vi "GOOP_VI_Item_OnCommand.vi"(10 "Command Tag":string, 11 "Object":u64) -> ()   [LabVIEW 2020]
uses:
  SubVIs/GOOP_ClassProviderClassType.ctl
  ClassProviders/Provider_BaseClassInterface/ClassWriter_class/ClassWriter.lvclass
  SubVIs/GOOP_UMLEditor_CallMainAction.ctl
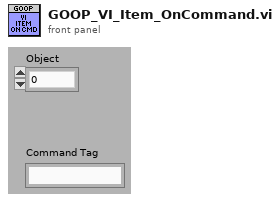
[diagram p1: front panel]
types:
  T1 = typedef "GOOP_ClassProviderClassType.ctl" = enum16{"ClassWriter", "ClassReader"}
  T2 = typedef "GOOP_UMLEditor_CallMainAction.ctl" = enum16{"OpenUmlEditor", "ReverseEngineering:WholeProject", "ReverseEngineering:OneClass", "ReverseEngineering:OneVI", "ShowInStateDiagram:OneVI", "OpenUMLFile"}
  T3 = typedef "ClassWriter.lvclass/RenameViOption.ctl" = cluster{"NewVIName":string, "VIs":path[], "IconOut":u8[][], "BgColor":u8}
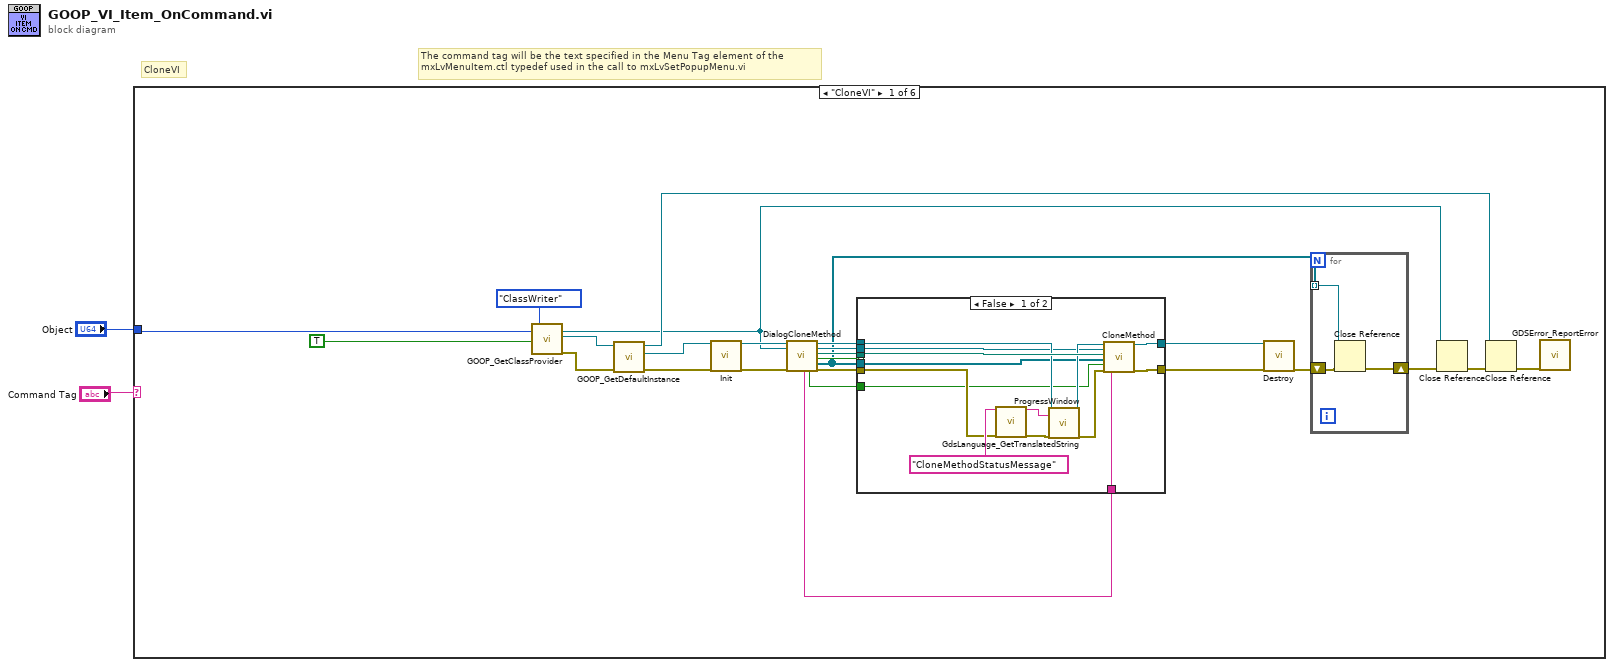
[diagram p0: block diagram]
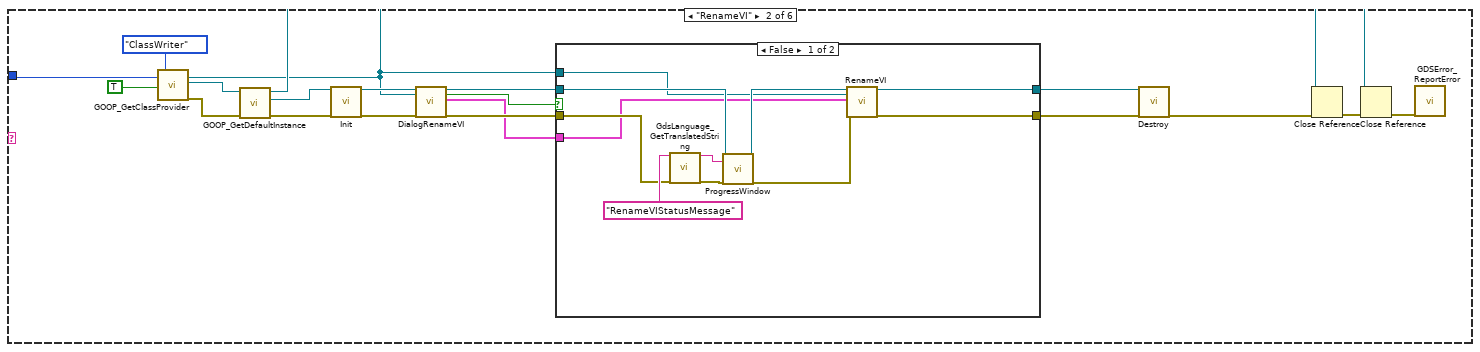
[diagram p3: hidden frame]
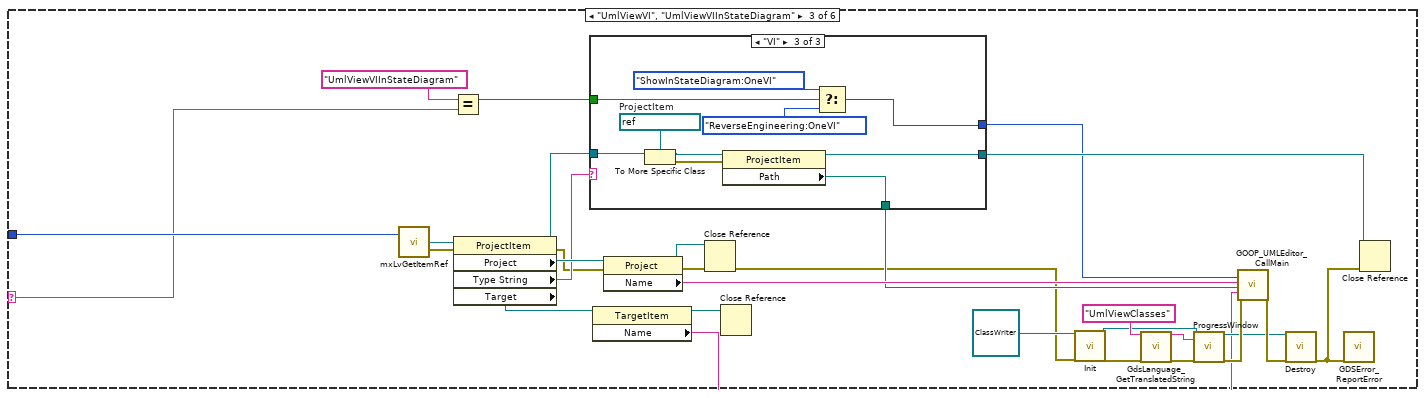
[diagram p5: hidden frame]
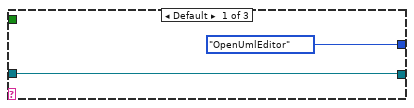
[diagram p6: hidden frame]
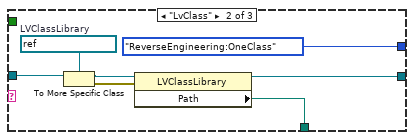
[diagram p7: hidden frame]
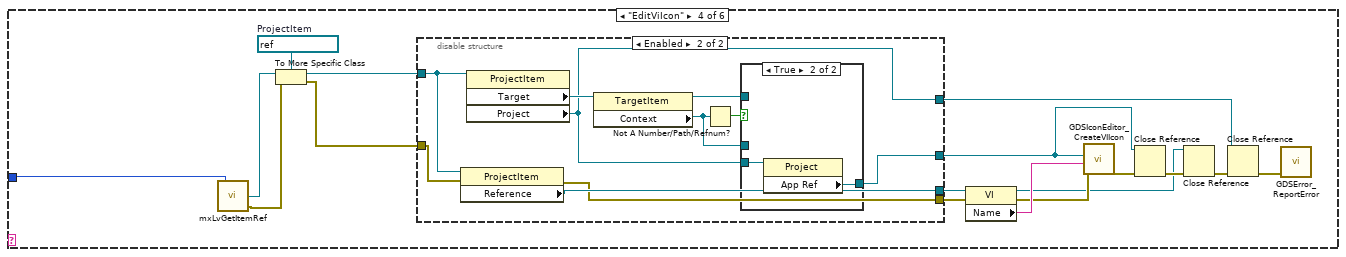
[diagram p8: hidden frame]
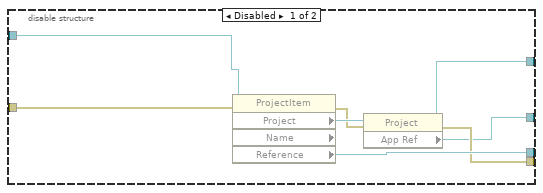
[diagram p9: hidden frame]
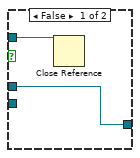
[diagram p10: hidden frame]
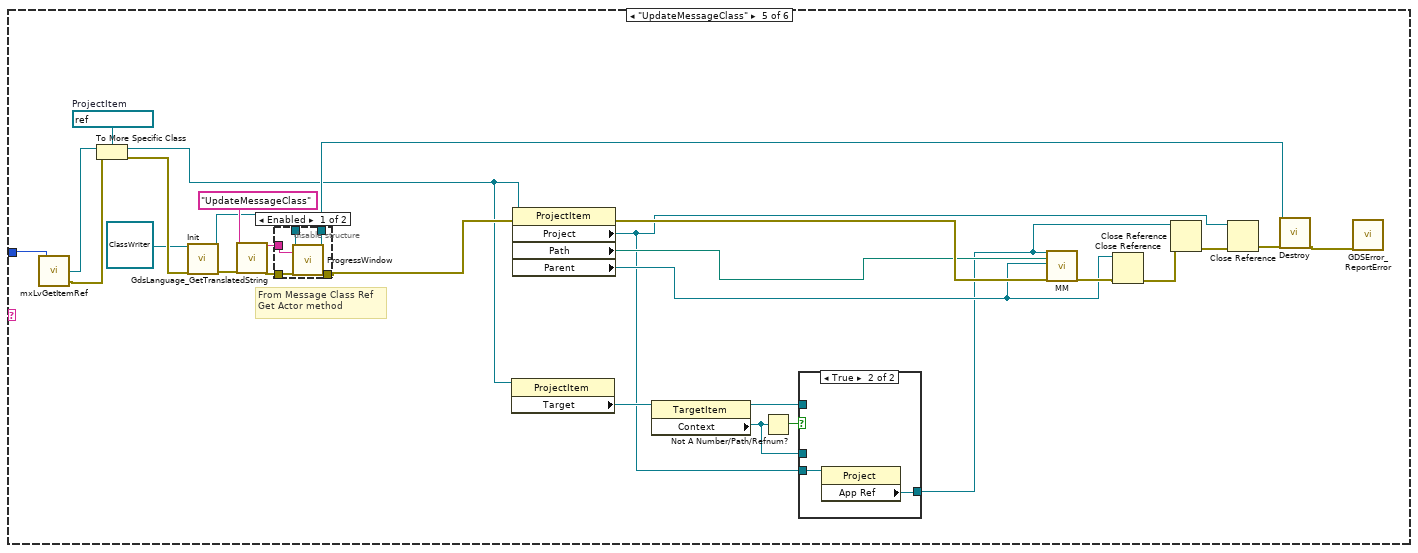
[diagram p11: hidden frame]
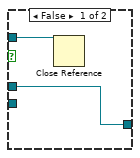
[diagram p12: hidden frame]
diagram:
  # "CloneVI"
  # "The command tag will be the text specified in the Menu Tag element of the \nmxLvMenuItem.ctl typedef used in the call to mxLvSetPopupMenu.vi"
  n1 = case shown="\"CloneVI\"" "Command Tag" {
    selector: "Command Tag" -> [_ _ w87 _ _ _]
    tunnel: "Object" -> [w24 w63 w89 w143 w193 _]
    frame "CloneVI" {
      n2 = call "GOOP_GetClassProvider.vi"("New Item Parent/Object"=w24, "CreateClass"=TRUE, "ProviderClassType"=GOOP_ClassProviderClassType."ClassWriter") -> ("ProjectItem"=w9:refnum<vi>, "LVClass.Open"=w22:refnum<vi>, "error out"=w23:errorcluster)  [unwired: 14 in]
      n3 = call "GOOP_GetDefaultInstance.vi"("error in"=w23, "LVClassIn"=w22) -> ("error out"=w20:errorcluster, "ClassWriter.lvclass"=w21:refnum<class "ClassWriter.lvclass">, "LVClassOut"=w19:refnum<vi>)  [unwired: 7 in]
      n4 = call-dynamic "Init.vi"("ClassWriter in"=w21, "error in (no error)"=w20) -> ("ClassWriter out"=w26:refnum<class "ClassWriter.lvclass">, "error out"=w25:errorcluster)  [unwired: 16 in]
      n5 = call-dynamic "DialogCloneMethod.vi"("ClassWriter.lvclass"=w26, "VIItemRefIn"=w9, "error in (no error)"=w25) -> ("NewVIDescriptionOut"=w3:string, "OpenAfter"=w4:bool, "ClassWriter.lvclassOut"=w17:refnum<class "ClassWriter.lvclass">, "VIItemRefOut"=w11:refnum<vi>, "NewVIPath"=w13:path, "Cancelled"=w14:bool, "LibraryOwners"=w6:refnum<vi>[], "error out"=w16:errorcluster)  [unwired: 9 in]
      n6 = case shown="False" w14 {
        tunnel: w17 -> [w37 w45]
        tunnel: w16 -> [w38 w46]
        tunnel: [w42 w46] -> w15
        tunnel: w13 -> [w44 _]
        tunnel: [w43 w45] -> w12
        tunnel: w6 -> [w34 _]
        tunnel: w11 -> [w33 _]
        tunnel: w4 -> [w32 _]
        tunnel: w3 -> [w31 _]
        frame False {
          n7 = call "GdsLanguage_GetTranslatedString.vi"("StringID(s)"="CloneMethodStatusMessage" ("Message(Exit)"), "error in (no error)"=w38) -> ("FirstStringOut"=w39:string, "error out"=w40:errorcluster)  [unwired: 14 in, 2 out]
          n8 = call-dynamic "ProgressWindow.vi"("ClassWriter in"=w37, "Message(Exit)"=w39, "error in (no error)"=w40) -> ("ClassWriter out"=w36:refnum<class "ClassWriter.lvclass">, "error out"=w35:errorcluster)  [unwired: 15 in]
          n9 = call-dynamic "CloneMethod.vi"("ClassWriter.lvclass"=w36, "VIItemRefIn"=w33, "NewVIPath"=w44, "LibraryOwners"=w34, "OpenVIWhenDone"=w32, "error in (no error)"=w35, "ViDescription"=w31) -> ("ClassWriter.lvclass"=w43:refnum<class "ClassWriter.lvclass">, "error out"=w42:errorcluster)  [unwired: 11 in]
        }
        frame True {
        }
      }
      n10 = call-dynamic "Destroy.vi"("ClassWriter.lvclass"=w12, "error in (no error)"=w15) -> ("error out"=w8:errorcluster)  [unwired: 17 in]
      n11 = for {
        shift-right: [w29] -> w7
        shift-left: w8 -> [w30]
        tunnel: w6 -> [w28] mode=indexing
        n12 = Close Reference(reference=w28, error in (no error)=w30) -> (error out=w29:errorcluster)
      }
      n13 = Close Reference(reference=w9, error in (no error)=w7) -> (error out=w10:errorcluster)
      n14 = Close Reference(reference=w19, error in (no error)=w10) -> (error out=w5:errorcluster)
      n15 = call "GDSError_ReportError.vi"("error in (no error)"=w5) -> ()  [unwired: 18 in, 1 out]
    }
    frame "RenameVI" {
      n16 = call "GOOP_GetClassProvider.vi"("New Item Parent/Object"=w63, "CreateClass"=TRUE, "ProviderClassType"=GOOP_ClassProviderClassType."ClassWriter") -> ("ProjectItem"=w47:refnum<vi>, "LVClass.Open"=w61:refnum<vi>, "error out"=w62:errorcluster)  [unwired: 14 in]
      n17 = call "GOOP_GetDefaultInstance.vi"("error in"=w62, "LVClassIn"=w61) -> ("error out"=w59:errorcluster, "ClassWriter.lvclass"=w60:refnum<class "ClassWriter.lvclass">, "LVClassOut"=w58:refnum<vi>)  [unwired: 7 in]
      n18 = call-dynamic "Init.vi"("ClassWriter in"=w60, "error in (no error)"=w59) -> ("ClassWriter out"=w65:refnum<class "ClassWriter.lvclass">, "error out"=w64:errorcluster)  [unwired: 16 in]
      n19 = call-dynamic "DialogRenameVI.vi"("ClassWriter.lvclass"=w65, "VIItemRefIn"=w47, "error in (no error)"=w64) -> ("ClassWriter.lvclassOut"=w56:refnum<class "ClassWriter.lvclass">, "Cancelled"=w49:bool, "RenameOption"=w48:T3, "error out"=w55:errorcluster)  [unwired: 13 in]
      n20 = case shown="False" w49 {
        tunnel: w56 -> [w71 w78]
        tunnel: w55 -> [w72 w79]
        tunnel: [w76 w79] -> w54
        tunnel: [w77 w78] -> w53
        tunnel: w48 -> [w67 _]
        tunnel: w47 -> [w68 _]
        frame False {
          n21 = call "GdsLanguage_GetTranslatedString.vi"("StringID(s)"="RenameVIStatusMessage" ("Message(Exit)"), "error in (no error)"=w72) -> ("FirstStringOut"=w73:string, "error out"=w74:errorcluster)  [unwired: 14 in, 2 out]
          n22 = call-dynamic "ProgressWindow.vi"("ClassWriter in"=w71, "Message(Exit)"=w73, "error in (no error)"=w74) -> ("ClassWriter out"=w70:refnum<class "ClassWriter.lvclass">, "error out"=w69:errorcluster)  [unwired: 15 in]
          n23 = call-dynamic "RenameVI.vi"("ObjectIn"=w70, "VIItemRefIn"=w68, "RenameOption"=w67, "error in (no error)"=w69) -> ("ObjectOut"=w77:refnum<class "ClassWriter.lvclass">, "error out"=w76:errorcluster)  [unwired: 14 in]
        }
        frame True {
        }
      }
      n24 = call-dynamic "Destroy.vi"("ClassWriter.lvclass"=w53, "error in (no error)"=w54) -> ("error out"=w51:errorcluster)  [unwired: 17 in]
      n25 = Close Reference(reference=w47, error in (no error)=w51) -> (error out=w52:errorcluster)
      n26 = Close Reference(reference=w58, error in (no error)=w52) -> (error out=w50:errorcluster)
      n27 = call "GDSError_ReportError.vi"("error in (no error)"=w50) -> ()  [unwired: 18 in, 1 out]
    }
    frame "UmlViewVI", "UmlViewVIInStateDiagram" {
      n28 = call <resource>:"mxLvGetItemRef.vi"("Item"=w89) -> ("Item Refnum"=w109:refnum<vi>, "error out"=w99:errorcluster)  [unwired: 1 in, 1 out]
      n29 = Equal?(x="UmlViewVIInStateDiagram", y=w87) -> (x = y?=w85:bool)
      n30 = property class="ProjectItem"(reference=w109, error in=w99) -> (reference out=w104:refnum<vi>, error out=w100:errorcluster, "Project"=w108:refnum<vi>, "Type String"=w102:string, "Target"=w81:refnum<vi>)
      n31 = case shown="\"VI\"" w102 {
        tunnel: w104 -> [w111 w118 w128]
        tunnel: [w111 w114 w124] -> w103
        tunnel: [_ w113 w123] -> w101
        tunnel: [GOOP_UMLEditor_CallMainAction."OpenUmlEditor" ("Enum") GOOP_UMLEditor_CallMainAction."ReverseEngineering:OneClass" ("Enum") w119] -> w88
        tunnel: w85 -> [_ _ w122]
        frame Default {
        }
        frame "LvClass" {
          w117 = refnum<vi> refnum  # LVClassLibrary
          n32 = To More Specific Class(target class=w117, reference=w118) -> (specific class reference=w116:refnum<vi>, error out=w115:errorcluster)  [unwired: 1 in]
          n33 = property class="LVClassLibrary"(reference=w116, error in=w115) -> (reference out=w114:refnum<vi>, "Path"=w113:path)  [unwired: 1 out]
        }
        frame "VI" {
          w127 = refnum<vi> refnum  # ProjectItem
          n34 = To More Specific Class(target class=w127, reference=w128) -> (specific class reference=w126:refnum<vi>, error out=w125:errorcluster)  [unwired: 1 in]
          n35 = property class="ProjectItem"(reference=w126, error in=w125) -> (reference out=w124:refnum<vi>, "Path"=w123:path)  [unwired: 1 out]
          n36 = Select(t=GOOP_UMLEditor_CallMainAction."ShowInStateDiagram:OneVI" ("Enum"), s=w122, f=GOOP_UMLEditor_CallMainAction."ReverseEngineering:OneVI" ("Enum")) -> (s? t:f=w119:T2)
        }
      }
      n37 = property class="TargetItem"(reference=w81) -> (reference out=w82:refnum<vi>, "Name"=w80:string)  [unwired: 1 in, 1 out]
      n38 = property class="Project"(reference=w108, error in=w100) -> (reference out=w105:refnum<vi>, error out=w106:errorcluster, "Name"=w107:string)
      n39 = Close Reference(reference=w105, error in (no error)=w106) -> (error out=w83:errorcluster)
      n40 = Close Reference(reference=w82) -> ()  [unwired: 1 in, 1 out]
      n41 = call-dynamic "Init.vi"("ClassWriter in"=refnum<class "ClassWriter.lvclass"> refnum, "error in (no error)"=w83) -> ("ClassWriter out"=w91:refnum<class "ClassWriter.lvclass">, "error out"=w95:errorcluster)  [unwired: 16 in]
      n42 = call "GdsLanguage_GetTranslatedString.vi"("StringID(s)"="UmlViewClasses" ("Message(Exit)"), "error in (no error)"=w95) -> ("FirstStringOut"=w98:string, "error out"=w97:errorcluster)  [unwired: 14 in, 2 out]
      n43 = call-dynamic "ProgressWindow.vi"("ClassWriter in"=w91, "Message(Exit)"=w98, "error in (no error)"=w97) -> ("ClassWriter out"=w92:refnum<class "ClassWriter.lvclass">, "error out"=w94:errorcluster)  [unwired: 15 in]
      n44 = call "GOOP_UMLEditor_CallMain.vi"("Enum"=w88, "Project"=w107, "Class/VI-Path"=w101, "Target"=w80, "error in (no error)"=w94) -> ("error out"=w93:errorcluster)  [unwired: 14 in]
      n45 = call-dynamic "Destroy.vi"("ClassWriter.lvclass"=w92, "error in (no error)"=w93) -> ("error out"=w84:errorcluster)  [unwired: 17 in]
      n46 = call "GDSError_ReportError.vi"("error in (no error)"=w84) -> ()  [unwired: 18 in, 1 out]
      n47 = Close Reference(reference=w103, error in (no error)=w84) -> ()  [unwired: 1 out]
    }
    frame "EditViIcon" {
      w145 = refnum<vi> refnum  # ProjectItem
      n48 = call <resource>:"mxLvGetItemRef.vi"("Item"=w143) -> ("Item Refnum"=w144:refnum<vi>, "error out"=w139:errorcluster)  [unwired: 1 in, 1 out]
      n49 = To More Specific Class(target class=w145, reference=w144, error in=w139) -> (specific class reference=w130:refnum<vi>, error out=w140:errorcluster)
      n50 = disable-structure shown="Enabled" {
        disable-tunnel: w140 -> [w153 w155]
        disable-tunnel: [w150 w154] -> w138
        disable-tunnel: [w149 w157] -> w135
        disable-tunnel: [w148 w156] -> w132
        disable-tunnel: w130 -> [w147 w158]
        disable-tunnel: [w146 w159] -> w129
        frame Disabled {
          n51 = property class="ProjectItem" props=["Project", "Name", "Reference"](reference=w147, error in=w153) -> (error out=w151:errorcluster, "Project"=w152:refnum<vi>, "Reference"=w149:refnum<vi>)  [unwired: 2 out]
          n52 = property class="Project"(reference=w152, error in=w151) -> (reference out=w150:refnum<vi>, error out=w148:errorcluster, "App Ref"=w146:refnum<vi>)
        }
        frame Enabled {
          n53 = property class="ProjectItem"(reference=w158, error in=w155) -> (error out=w156:errorcluster, "Reference"=w157:refnum<vi>)  [unwired: 1 out]
          n54 = property class="ProjectItem"(reference=w158) -> ("Target"=w160:refnum<vi>, "Project"=w154:refnum<vi>)  [unwired: 1 in, 2 out]
          n55 = property class="TargetItem"(reference=w160) -> (reference out=w163:refnum<vi>, "Context"=w162:refnum<vi>)  [unwired: 1 in, 1 out]
          n56 = Not A Number/Path/Refnum?(number/path/refnum=w162) -> (NaN/Path/Refnum?=w161:bool)
          n57 = case shown="True" w161 {
            tunnel: [w165 w167] -> w159
            tunnel: w154 -> [_ w166]
            tunnel: w162 -> [w165 _]
            tunnel: w163 -> [w164 _]
            frame False {
              n58 = Close Reference(reference=w164) -> ()  [unwired: 1 in, 1 out]
            }
            frame True {
              n59 = property class="Project"(reference=w166) -> ("App Ref"=w167:refnum<vi>)  [unwired: 1 in, 2 out]
            }
          }
        }
      }
      n60 = property class="VI"(reference=w135, error in=w132) -> (reference out=w131:refnum<vi>, error out=w133:errorcluster, "Name"=w134:string)
      n61 = call "GDSIconEditor_CreateVIIcon.vi"("error in (no error)"=w133, "Application:Menu Launch:VI"=w134, "Application:Menu Launch:App"=w129) -> ("error out"=w137:errorcluster)  [unwired: 8 in]
      n62 = Close Reference(reference=w129, error in (no error)=w137) -> (error out=w136:errorcluster)
      n63 = Close Reference(reference=w131, error in (no error)=w136) -> (error out=w142:errorcluster)
      n64 = Close Reference(reference=w138, error in (no error)=w142) -> (error out=w141:errorcluster)
      n65 = call "GDSError_ReportError.vi"("error in (no error)"=w141) -> ()  [unwired: 18 in, 1 out]
    }
    frame "UpdateMessageClass" {
      w195 = refnum<vi> refnum  # ProjectItem
      # "From Message Class Ref\nGet Actor method"
      n66 = call <resource>:"mxLvGetItemRef.vi"("Item"=w193) -> ("Item Refnum"=w194:refnum<vi>, "error out"=w192:errorcluster)  [unwired: 1 in, 1 out]
      n67 = To More Specific Class(target class=w195, reference=w194, error in=w192) -> (specific class reference=w170:refnum<vi>, error out=w183:errorcluster)
      n68 = call-dynamic "Init.vi"("ClassWriter in"=refnum<class "ClassWriter.lvclass"> refnum, "error in (no error)"=w183) -> ("ClassWriter out"=w184:refnum<class "ClassWriter.lvclass">, "error out"=w186:errorcluster)  [unwired: 16 in]
      n69 = call "GdsLanguage_GetTranslatedString.vi"("StringID(s)"="UpdateMessageClass" ("Message(Exit)"), "error in (no error)"=w186) -> ("FirstStringOut"=w187:string, "error out"=w185:errorcluster)  [unwired: 14 in, 2 out]
      n70 = disable-structure shown="Enabled" {
        disable-tunnel: w187 -> [w204 _]
        disable-tunnel: [w203 w206] -> w181
        disable-tunnel: w185 -> [w202 w206]
        disable-tunnel: w184 -> [w201 w205]
        disable-tunnel: [w200 w205] -> w178
        frame Enabled {
          n71 = call-dynamic "ProgressWindow.vi"("ClassWriter in"=w201, "Message(Exit)"=w204, "error in (no error)"=w202) -> ("ClassWriter out"=w200:refnum<class "ClassWriter.lvclass">, "error out"=w203:errorcluster)  [unwired: 15 in]
        }
        frame Disabled {
        }
      }
      n72 = property class="ProjectItem"(reference=w170) -> ("Target"=w171:refnum<vi>)  [unwired: 1 in, 2 out]
      n73 = property class="ProjectItem"(reference=w170, error in=w181) -> (error out=w191:errorcluster, "Project"=w168:refnum<vi>, "Path"=w190:path, "Parent"=w175:refnum<vi>)  [unwired: 1 out]
      n74 = property class="TargetItem"(reference=w171) -> (reference out=w174:refnum<vi>, "Context"=w173:refnum<vi>)  [unwired: 1 in, 1 out]
      n75 = Not A Number/Path/Refnum?(number/path/refnum=w173) -> (NaN/Path/Refnum?=w172:bool)
      n76 = case shown="True" w172 {
        tunnel: [w197 w199] -> w169
        tunnel: w168 -> [_ w198]
        tunnel: w173 -> [w197 _]
        tunnel: w174 -> [w196 _]
        frame False {
          n77 = Close Reference(reference=w196) -> ()  [unwired: 1 in, 1 out]
        }
        frame True {
          n78 = property class="Project"(reference=w198) -> ("App Ref"=w199:refnum<vi>)  [unwired: 1 in, 2 out]
        }
      }
      n79 = call "MM.vi"("AppInst"=w169, "ActorMethod"=w190, "ActorClassItemRef(Don't Delete)"=w175, "error in"=w191) -> ("error out"=w177:errorcluster)  [unwired: 15 in]
      n80 = Close Reference(reference=w175, error in (no error)=w177) -> (error out=w176:errorcluster)
      n81 = Close Reference(reference=w169, error in (no error)=w176) -> (error out=w189:errorcluster)
      n82 = Close Reference(reference=w168, error in (no error)=w189) -> (error out=w180:errorcluster)
      n83 = call-dynamic "Destroy.vi"("ClassWriter.lvclass"=w178, "error in (no error)"=w180) -> ("error out"=w179:errorcluster)  [unwired: 17 in]
      n84 = call "GDSError_ReportError.vi"("error in (no error)"=w179) -> ()  [unwired: 18 in, 1 out]
    }
    frame Default {
    }
  }
